vi "home_single_channel.vi"() -> (1 "Sensor Sampling":waveform(dbl)[](graph))   [LabVIEW 2020]
uses:
  C:/Users/359167/Documents/LabVIEW_ws/Thorlabs.MotionControl.DeviceManagerCLI.dll
  Thorlabs.MotionControl.DeviceManagerCLI.dll
  C:/Users/359167/Documents/LabVIEW_ws/Thorlabs.MotionControl.KCube.InertialMotorCLI.dll
  Thorlabs.MotionControl.KCube.InertialMotorCLI.dll
  <vilib>/DAQmx/read.llb/DAQmx Read (Analog 1D Wfm NChan NSamp).vi
  <vilib>/Analysis/baseanly.llb/Mean (DBL).vi
  <vilib>/DAQmx/create/channels.llb/DAQmx Create Channel (AI-Voltage-Basic).vi
  <vilib>/DAQmx/configure/timing.llb/DAQmx Timing (Sample Clock).vi
  <vilib>/DAQmx/miscellaneous.llb/DAQmx Fill In Error Info.vi
  <vilib>/Utility/file.llb/Write Delimited Spreadsheet (DBL).vi
  <vilib>/Analysis/NI_AALBase.lvlib
panel:
  out "32bit integer":i32
  out "Loop Change":dbl
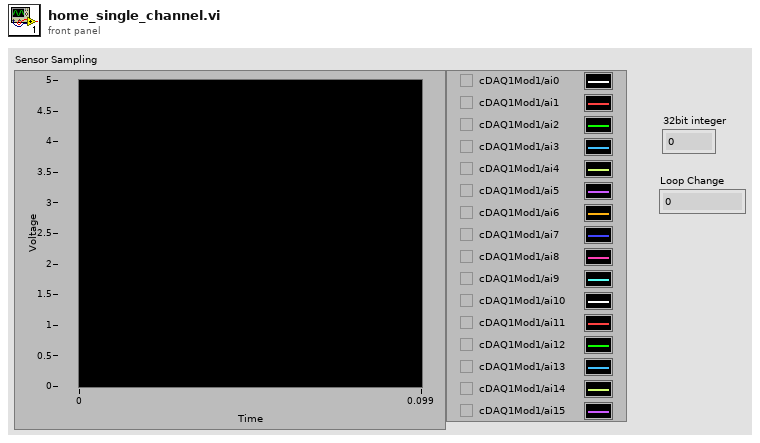
[diagram p1: front panel]
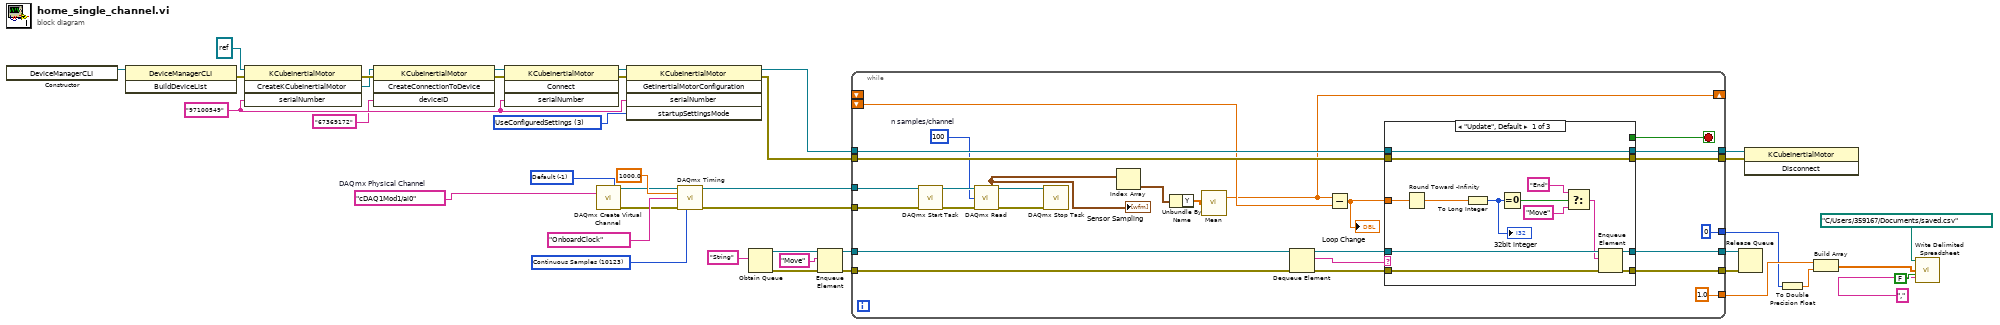
[diagram p0: block diagram]
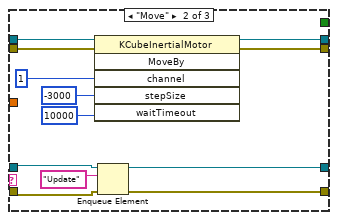
[diagram p2: hidden frame]
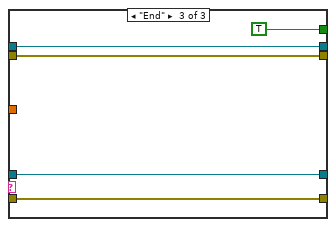
[diagram p3: hidden frame]
diagram:
  w7 = "97100549" ("SerialNumber")
  w12 = 3 items=["UseDeviceSettings"=1, "UseFileSettings"=2, "UseConfiguredSettings"=3] ("startupSettingsMode")
  w24 = tag "cDAQ1Mod1/ai0"  # DAQmx Physical Channel
  w29 = -1 items=["Default"=-1, "RSE"=10083, "NRSE"=10078, "Differential"=10106, "Pseudodifferential"=12529] ("input terminal configuration")
  w30 = 10123 items=["Finite Samples"=10178, "Continuous Samples"=10123, "Hardware Timed Single Point"=12522] ("sample mode")
  n1 = constructor class="DeviceManagerCLI"() -> (reference out=w16:refnum<k24>)  [unwired: 3 in, 2 out]
  n2 = invoke class="DeviceManagerCLI" method="BuildDeviceList"(reference=w16) -> (error out=w14:errorcluster)  [unwired: 2 in, 2 out]
  n3 = invoke class="KCubeInertialMotor" method="CreateKCubeInertialMotor"(reference=refnum<k24> refnum, error in=w14, "serialNumber"=w7) -> (error out=w13:errorcluster, "CreateKCubeInertialMotor"=w6:refnum<k24>)  [unwired: 1 in, 2 out]
  n4 = invoke class="KCubeInertialMotor" method="CreateConnectionToDevice"(reference=w6, error in=w13, "deviceID"="67369172") -> (reference out=w11:refnum<k24>, error out=w10:errorcluster)  [unwired: 1 in, 2 out]
  n5 = invoke class="KCubeInertialMotor" method="Connect"(reference=w11, error in=w10, "serialNumber"=w7) -> (reference out=w9:refnum<k24>, error out=w8:errorcluster)  [unwired: 1 in, 2 out]
  n6 = call-poly <vilib>:"DAQmx Create Virtual Channel.vi"("input terminal configuration"=w29, "physical channels"=w24) -> ("task out"=w25:refnum<k21>, "error out"=w26:errorcluster)  [unwired: 12 in]
  n7 = invoke class="KCubeInertialMotor" method="GetInertialMotorConfiguration"(reference=w9, error in=w8, "serialNumber"=w7, "startupSettingsMode"=w12) -> (reference out=w3:refnum<k24>, error out=w4:errorcluster)  [unwired: 1 in, 3 out]
  n8 = call-poly <vilib>:"DAQmx Timing.vi"("task/channels in"=w25, "sample mode"=w30, "rate"=1000.0 ("sample rate"), "source"=tag "OnboardClock", "error in"=w26) -> ("task out"=w2:refnum<k21>, "error out"=w1:errorcluster)  [unwired: 9 in]
  n9 = Obtain Queue(element data type="String") -> (queue out=w34:refnum<queue>, error out=w33:errorcluster)  [unwired: 4 in, 1 out]
  n10 = Enqueue Element(queue=w34, element="Move", error in (no error)=w33) -> (queue out=w32:refnum<queue>, error out=w31:errorcluster)  [unwired: 1 in, 1 out]
  n11 = while {
    shift-right: [w43] -> _
    shift-left: _ -> [_]
    tunnel: [w60] -> w39
    tunnel: [w61] -> w38
    tunnel: w3 -> [w63]
    tunnel: w4 -> [w62]
    tunnel: w31 -> [w49]
    tunnel: [w59] -> w37
    tunnel: [w51] -> w36
    tunnel: w32 -> [w50]
    shift-left: _ -> [w44]
    tunnel: [0] -> w17
    tunnel: [1.0] -> w19
    tunnel: w2 -> [w42]
    tunnel: w1 -> [w41]
    stop <- w65 stop-if-true
    w54 = 100  # n samples/channel
    # "Consumer"
    n12 = call <vilib>:"DAQmx Start Task.vi"("task/channels in"=w42, "error in"=w41) -> ("task out"=w55:refnum<k21>, "error out"=w56:errorcluster)  [unwired: 12 in]
    n13 = call-poly <vilib>:"DAQmx Read.vi"("task/channels in"=w55, "number of samples per channel"=w54, "error in"=w56) -> ("data"=w48:waveform(dbl)[], "task out"=w57:refnum<k21>, "error out"=w58:errorcluster)  [unwired: 10 in]
    "Sensor Sampling" <- w48
    n14 = call <vilib>:"DAQmx Stop Task.vi"("task/channels in"=w57, "error in"=w58) -> ()  [unwired: 12 in, 2 out]
    n15 = Index Array(array=w48) -> (element=w53:waveform(dbl))  [unwired: 1 in]
    n16 = Unbundle By Name(w53) -> ("Y"=w52:dbl[])
    n17 = call-poly <vilib>:"Mean.vi"("X"=w52) -> ("mean"=w43:dbl)  [unwired: 1 out]
    n18 = Dequeue Element(queue=w50, error in (no error)=w49) -> (queue out=w67:refnum<queue>, element=w66:string, error out=w64:errorcluster)  [unwired: 1 in, 1 out]
    n19 = Subtract(x=w43, y=w44) -> (x-y=w47:dbl)
    "Loop Change" <- w47
    n20 = case shown="\"Update\", Default" w66 {
      tunnel: w67 -> [w78 w88 w93]
      tunnel: [w80 w86 w94] -> w59
      tunnel: [_ _ TRUE] -> w65
      tunnel: w64 -> [w79 w87 w94]
      tunnel: w62 -> [w76 w92 w96]
      tunnel: [w77 w91 w95] -> w61
      tunnel: [w76 w90 w96] -> w60
      tunnel: w63 -> [w77 w89 w95]
      tunnel: [w75 w85 w93] -> w51
      tunnel: w47 -> [w68 _ _]
      frame "Update", Default {
        n21 = Round Toward -Infinity(1:w68) -> (0:w69:dbl)
        n22 = To Long Integer(number=w69) -> (32bit integer=w70:i32)
        "32bit integer" <- w70
        n23 = Equal To 0?(x=w70) -> (x = 0?=w74:bool)
        n24 = Select(t="End", s=w74, f="Move" ("element")) -> (s? t:f=w71:string)
        n25 = Enqueue Element(queue=w78, element=w71, error in (no error)=w79) -> (queue out=w75:refnum<queue>, error out=w80:errorcluster)  [unwired: 1 in, 1 out]
      }
      frame "Move" {
        n26 = invoke class="KCubeInertialMotor" method="MoveBy"(reference=w89, error in=w92, "channel"=1 ("Channel"), "stepSize"=-3000, "waitTimeout"=10000) -> (reference out=w91:refnum<k24>, error out=w90:errorcluster)  [unwired: 1 in, 4 out]
        n27 = Enqueue Element(queue=w88, element="Update", error in (no error)=w87) -> (queue out=w85:refnum<queue>, error out=w86:errorcluster)  [unwired: 1 in, 1 out]
      }
      frame "End" {
      }
    }
  }
  n28 = Release Queue(queue=w36, error in (no error)=w37) -> ()  [unwired: 1 in, 3 out]
  n29 = invoke class="KCubeInertialMotor" method="Disconnect"(reference=w38, error in=w39) -> ()  [unwired: 1 in, 3 out]
  n30 = To Double Precision Float(number=w17) -> (double precision float=w18:dbl)
  n31 = Build Array(w19, w18) -> (w20:dbl[])
  n32 = call-poly <vilib>:"Write Delimited Spreadsheet.vi"("file path (dialog if empty)"=path "C:/Users/359167/Documents/saved.csv" ("Path"), "1D data"=w20, "append to file? (new file:F)"=FALSE, "delimiter (\\t)"="," ("delimiter (\\t)")) -> ()  [unwired: 10 in, 2 out]
